vi "Validar MCU.vi"(11 "Dato_Recibido":string) -> (3 "Dato_OK":string)   [LabVIEW 2019]
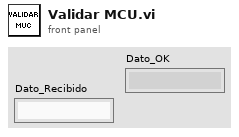
[diagram p1: front panel]
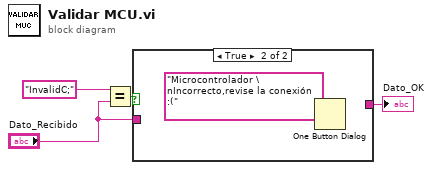
[diagram p0: block diagram]
diagram:
  n1 = Equal?(x="InvalidC;", y="Dato_Recibido") -> (x = y?=w4:bool)
  n2 = case shown="True" w4 {
    tunnel: [w5 _] -> w1
    tunnel: "Dato_Recibido" -> [w5 _]
    frame False {
    }
    frame True {
      n3 = One Button Dialog(message="Microcontrolador \nIncorrecto,revise la conexión :(") -> ()  [unwired: 1 in, 1 out]
    }
  }
  "Dato_OK" <- w1
